vi "home.vi"(1 "速度":dbl, 2 "连接ID":refnum<k5>) -> (0 "连接ID":refnum<k5>)   [LabVIEW 2017]
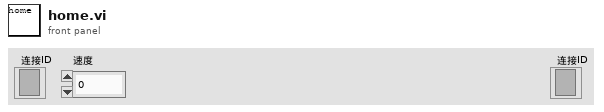
[diagram p1: front panel]
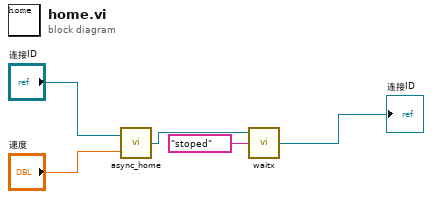
[diagram p0: block diagram]
diagram:
  n1 = call "async_home.vi"("velocity"="速度", "连接ID"="连接ID") -> ("连接ID输出"=w3:refnum<k5>)
  n2 = call "waitx.vi"("String Value"="stoped", "连接ID"=w3) -> ("连接ID 2"=→"连接ID":refnum<k5>)  [unwired: 1 in]
